vi "ADC_segment.vi"(0 "First point":i32, 1 "Segment Number":i32, 2 "Segment Length":i32, 3 "Segment Period":dbl, 4 "data in":dbl[][](array[numeric])) -> (5 "data out":dbl[][](array[numeric]))   [LabVIEW 2013]
uses:
  <vilib>/Analysis/baseanly.llb/Mean (DBL).vi
  <vilib>/Analysis/NI_AALBase.lvlib
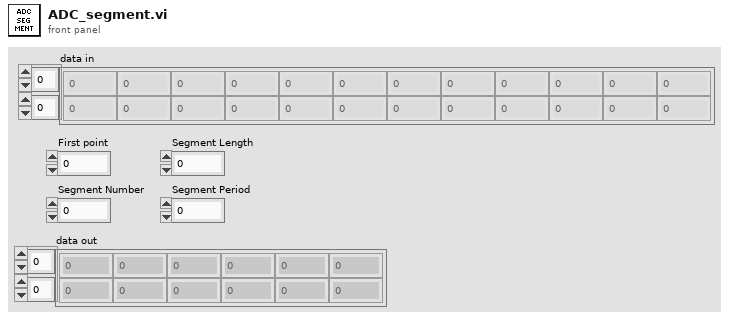
[diagram p1: front panel]
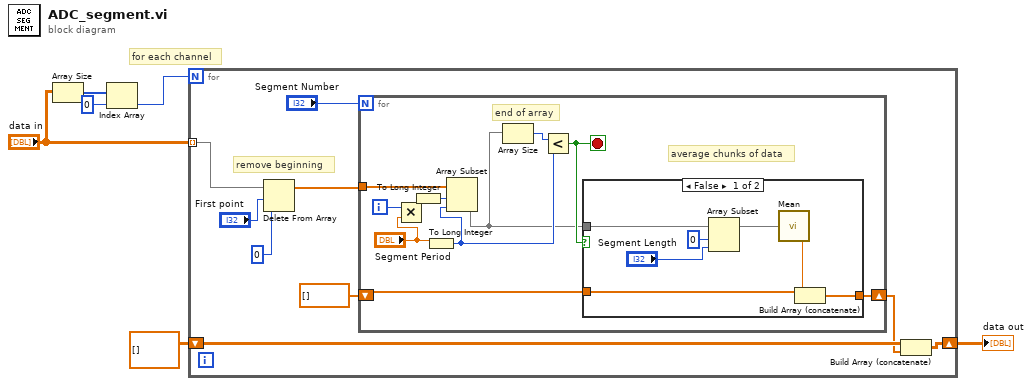
[diagram p0: block diagram]
diagram:
  # "for each channel"
  n1 = Array Size(array="data in") -> (size(s)=w1:i32[])
  n2 = Index Array(array=w1, index=0) -> (element=w2:i32)
  n3 = for {
    N: w2 -> [_]
    tunnel: "data in" -> [w10] mode=indexing
    shift-right: [w14] -> w6
    shift-left: dbl[][] [] -> [w15]
    # "remove beginning"
    n4 = Delete From Array(array=w10, length="First point", index=0) -> (array with subset deleted=w11:dbl[])  [unwired: 1 out]
    n5 = for {
      N: "Segment Number" -> [_]
      shift-right: [w25] -> w13
      shift-left: dbl[] [] -> [w26]
      tunnel: w11 -> [w23]
      i -> [w22]
      stop <- w17 stop-if-true
      # "end of array"
      # "average chunks of data"
      n6 = Multiply(x=w22, y="Segment Period") -> (x*y=w20:dbl)
      n7 = To Long Integer(number=w20) -> (32bit integer=w19:i32)
      n8 = To Long Integer(number="Segment Period") -> (32bit integer=w18:i32)
      n9 = Array Subset(array=w23, index=w19, length=w18) -> (w16:dbl[])
      n10 = Array Size(array=w16) -> (size(s)=w24:i32)
      n11 = Less?(x=w24, y=w18) -> (x < y?=w17:bool)
      n12 = case shown="False" w17 {
        tunnel: w16 -> [w33 _]
        tunnel: w26 -> [w32 w34]
        tunnel: [w31 w34] -> w25
        frame False {
          n13 = Array Subset(array=w33, index=0, length="Segment Length") -> (w29:dbl[])
          n14 = call-poly <vilib>:"Mean.vi"("X"=w29) -> ("mean"=w30:dbl)  [unwired: 1 out]
          n15 = Build Array (concatenate)(w32, w30) -> (w31:dbl[])
        }
        frame True {
        }
      }
    }
    n16 = Build Array (concatenate)(w15, w13) -> (w14:dbl[][])
  }
  "data out" <- w6
